vi "Hold_Galvos_Run_Camera.vi"() -> ()   [LabVIEW 2017]
doc: "This example demonstrates how to continuously generate digital pulses using a counter output."
uses:
  <vilib>/Utility/error.llb/DialogType.ctl
  <vilib>/DAQmx/write.llb/DAQmx Write (Analog 1D DBL NChan 1Samp).vi
  <vilib>/DAQmx/create/channels.llb/DAQmx Create Channel (AO-Voltage-Basic).vi
  <vilib>/DAQmx/create/channels.llb/DAQmx Create Channel (CO-Pulse Generation-Frequency).vi
  <vilib>/DAQmx/configure/timing.llb/DAQmx Timing (Implicit).vi
  <vilib>/DAQmx/miscellaneous.llb/DAQmx Fill In Error Info.vi
  <resource>/objmgr/daqmx.rc
panel:
  in  "Galvo analog output channel(s)":tag="Dev1/ao0:1"
  out "Interface Name":string="img0"
  out "Image":T1(plugin-control)
  out "Frame Rate (Hz)":dbl
  out "Actual Duty Cycle":dbl
  out "Actual Frequency":dbl
  in  "Duty Cycle (%)":dbl=95.0 format="%.6f"
  in  "Frequency (kHz)":dbl=130.0 format="%.6f"
  in  "Output Terminal":tag="/Dev1/PFI2"
  in  "Stop":bool
  in  "Counter":tag="Dev1/ctr0"
  # "Channel Settings"
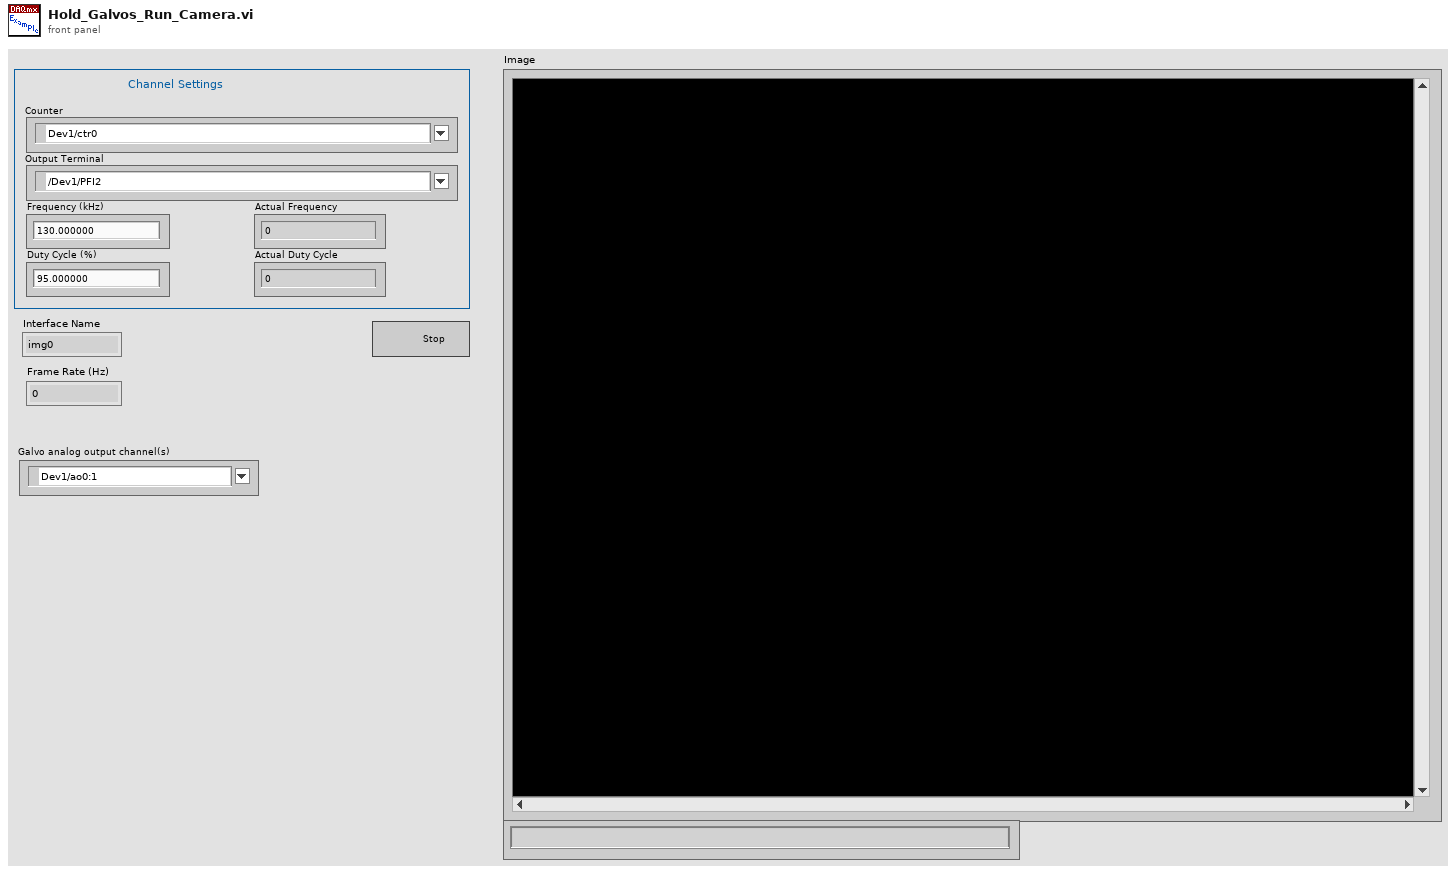
[diagram p1: front panel]
types:
  T1 = typedef "IMAQ Image.ctl" = refnum<image>
  T2 = typedef "DialogType.ctl" = u16
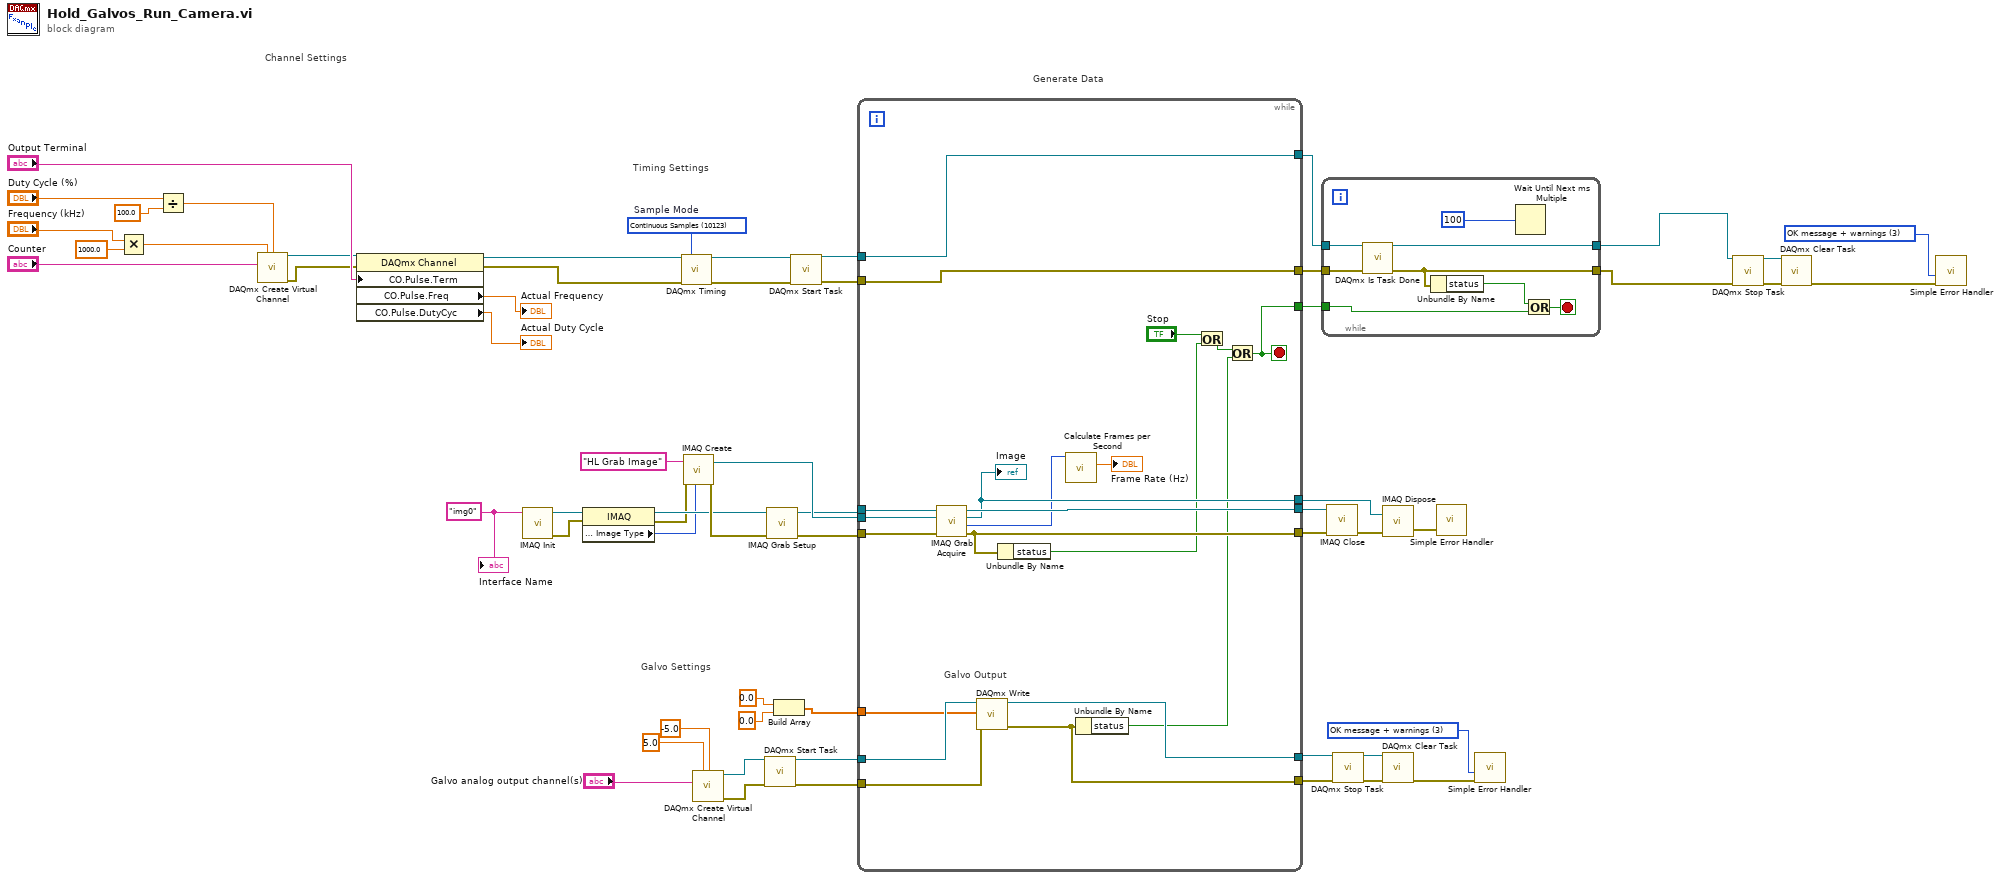
[diagram p0: block diagram]
diagram:
  w21 = T2 3 items=["no dialog", "OK message", "continue or stop message", "OK message + warnings", "continue/stop + warnings"] ("type of dialog (OK msg:1)")
  w30 = 10123 items=["Finite Samples"=10178, "Continuous Samples"=10123, "Hardware Timed Single Point"=12522]  # Sample Mode
  w50 = "img0" ("Interface Name")
  w57 = T2 3 items=["no dialog", "OK message", "continue or stop message", "OK message + warnings", "continue/stop + warnings"] ("type of dialog (OK msg:1)")
  # "Generate Data"
  # "Galvo Settings"
  # "Timing Settings"
  # "Channel Settings"
  n1 = Multiply(x="Frequency (kHz)", y=1000.0) -> (x*y=w9:dbl)
  n2 = Divide(x="Duty Cycle (%)", y=100.0) -> (x/y=w7:dbl)
  n3 = call-poly <vilib>:"DAQmx Create Virtual Channel.vi"("frequency"=w9, "duty cycle"=w7, "counter"="Counter") -> ("task out"=w34:refnum<k21>, "error out"=w35:errorcluster)  [unwired: 11 in]
  n4 = property class="DAQmx Channel"(reference=w34, error in=w35, "CO.Pulse.Term"="Output Terminal") -> (reference out=w38:refnum<k21>, error out=w37:errorcluster, "CO.Pulse.Freq"=→"Actual Frequency":dbl, "CO.Pulse.DutyCyc"=→"Actual Duty Cycle":dbl)
  n5 = call <vilib>:"IMAQ Init.vi"("Interface Name"=w50) -> ("error out"=w48:errorcluster, "IMAQ Session Out"=w49:refnum<k11>)  [unwired: 1 in, 8 out]
  n6 = property class="IMAQ"(reference=w49, error in=w48) -> (reference out=w47:refnum<k11>, error out=w46:errorcluster, "Image Parameters : Image Type"=w45:u32)
  n7 = call-poly <vilib>:"DAQmx Timing.vi"("task/channels in"=w38, "sample mode"=w30, "error in"=w37) -> ("task out"=w33:refnum<k21>, "error out"=w32:errorcluster)  [unwired: 11 in]
  n8 = call "IMAQ Create"("Image Name"="HL Grab Image", "Image Type"=w45, "error in (no error)"=w46) -> ("New Image"=w43:T1, "error out"=w51:errorcluster)  [unwired: 1 in, 1 out]
  n9 = call-poly <vilib>:"DAQmx Create Virtual Channel.vi"("maximum value"=5.0 ("Max Voltage"), "minimum value"=-5.0 ("Min Voltage"), "physical channels"="Galvo analog output channel(s)") -> ("task out"=w25:refnum<k21>, "error out"=w24:errorcluster)  [unwired: 11 in]
  n10 = call <vilib>:"DAQmx Start Task.vi"("task/channels in"=w25, "error in"=w24) -> ("task out"=w18:refnum<k21>, "error out"=w17:errorcluster)  [unwired: 12 in]
  n11 = call <vilib>:"IMAQ Grab Setup.vi"("error in (no error)"=w51, "IMAQ Session In"=w47) -> ("error out"=w42:errorcluster, "IMAQ Session Out"=w41:refnum<k11>)  [unwired: 8 out]
  n12 = Build Array(0.0 ("X (V)"), 0.0 ("Y (V)")) -> (w12:dbl[])
  n13 = call <vilib>:"DAQmx Start Task.vi"("task/channels in"=w33, "error in"=w32) -> ("task out"=w29:refnum<k21>, "error out"=w28:errorcluster)  [unwired: 12 in]
  n14 = while {
    tunnel: [w80] -> w54
    tunnel: [w79] -> w53
    tunnel: [w78] -> w52
    tunnel: w43 -> [w74]
    tunnel: w42 -> [w73]
    tunnel: w41 -> [w72]
    tunnel: w29 -> [w64]
    tunnel: w28 -> [w63]
    tunnel: w18 -> [w71]
    tunnel: w17 -> [w70]
    tunnel: [w69] -> w16
    tunnel: [w68] -> w15
    tunnel: w12 -> [w65]
    tunnel: [w64] -> w5
    tunnel: [w63] -> w4
    tunnel: [w61] -> w1
    stop <- w61 stop-if-true
    # "Galvo Output"
    n15 = call <vilib>:"IMAQ Grab Acquire.vi"("error in (no error)"=w73, "Image In"=w74, "IMAQ Session In"=w72) -> ("error out"=w80:errorcluster, "Acquired Buffer Number"=w77:u32, "Image Out"=w78:T1, "IMAQ Session Out"=w79:refnum<k11>)  [unwired: 1 in, 4 out]
    "Image" <- w78
    n16 = call-poly <vilib>:"DAQmx Write.vi"("task/channels in"=w71, "data"=w65, "error in"=w70) -> ("task out"=w69:refnum<k21>, "error out"=w68:errorcluster)  [unwired: 10 in, 1 out]
    n17 = Unbundle By Name(w80) -> ("status"=w75:bool)
    n18 = call <vilib>:"Calculate Frames per Second.vi"("Buffer Number"=w77) -> ("Processed Frames/s"=→"Frame Rate (Hz)":dbl)  [unwired: 8 in, 2 out]
    n19 = Unbundle By Name(w68) -> ("status"=w66:bool)
    n20 = Or(x="Stop", y=w75) -> (x .or. y?=w67:bool)
    n21 = Or(x=w67, y=w66) -> (x .or. y?=w61:bool)
  }
  n22 = while {
    tunnel: w5 -> [w88]
    tunnel: w4 -> [w87]
    tunnel: [w84] -> w2
    tunnel: [w85] -> w3
    tunnel: w1 -> [w81]
    stop <- w86 stop-if-true
    n23 = call <vilib>:"DAQmx Is Task Done.vi"("task/channels in"=w88, "error in"=w87) -> ("task out"=w85:refnum<k21>, "error out"=w84:errorcluster)  [unwired: 11 in, 1 out]
    n24 = Unbundle By Name(w84) -> ("status"=w83:bool)
    n25 = Wait Until Next ms Multiple(millisecond multiple=u32 100) -> ()  [unwired: 1 out]
    n26 = Or(x=w83, y=w81) -> (x .or. y?=w86:bool)
  }
  n27 = call <vilib>:"IMAQ Close.vi"("error in (no error)"=w54, "IMAQ Session In"=w53) -> ("error out"=w56:errorcluster)  [unwired: 9 out]
  n28 = call <vilib>:"DAQmx Stop Task.vi"("task/channels in"=w16, "error in"=w15) -> ("task out"=w23:refnum<k21>, "error out"=w22:errorcluster)  [unwired: 12 in]
  n29 = call "IMAQ Dispose"("Image"=w52, "error in (no error)"=w56) -> ("error out"=w55:errorcluster)  [unwired: 1 in, 3 out]
  n30 = call <vilib>:"DAQmx Clear Task.vi"("task in"=w23, "error in"=w22) -> ("error out"=w27:errorcluster)  [unwired: 13 in]
  n31 = call <vilib>:"Simple Error Handler.vi"("error in (no error)"=w55) -> ()  [unwired: 1 in, 8 out]
  n32 = call <vilib>:"Simple Error Handler.vi"("type of dialog (OK msg:1)"=w21, "error in (no error)"=w27) -> ()  [unwired: 3 in, 5 out]
  n33 = call <vilib>:"DAQmx Stop Task.vi"("task/channels in"=w3, "error in"=w2) -> ("task out"=w59:refnum<k21>, "error out"=w58:errorcluster)  [unwired: 12 in]
  n34 = call <vilib>:"DAQmx Clear Task.vi"("task in"=w59, "error in"=w58) -> ("error out"=w60:errorcluster)  [unwired: 13 in]
  n35 = call <vilib>:"Simple Error Handler.vi"("type of dialog (OK msg:1)"=w57, "error in (no error)"=w60) -> ()  [unwired: 3 in, 5 out]
  "Interface Name" <- w50
